vi "Felix Event FSM Producer-Consumer Template.vi"() -> ()   [LabVIEW 2017]
uses:
  FSM Queue Datatype.ctl
panel:
  out "starat seq 2 argument":dbl
  in  "Seq 2 argument":dbl format="%#_13g"
  in  "Loop Back":bool
  in  "Skip Step 2":bool
  out "FSM State":string
  out "LED 2.3":bool
  out "LED 2.2":bool
  out "LED 2.1":bool
  out "LED 1.3":bool
  out "LED 1.2":bool
  out "LED 1.1":bool
  in  "Start Sequence 2":bool
  in  "Start Sequence 1":bool
  in  "stop":bool
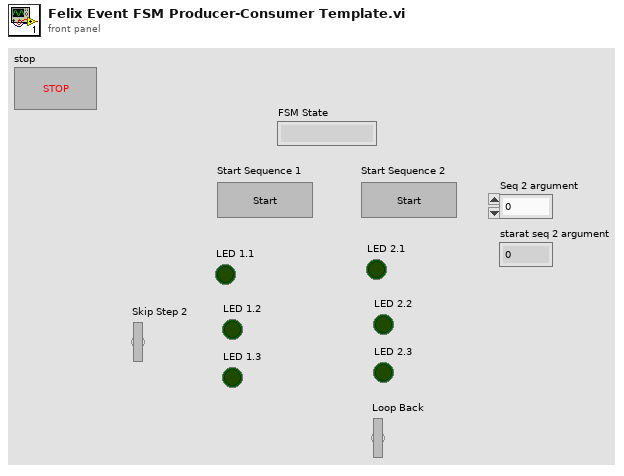
[diagram p1: front panel]
types:
  T1 = cluster{"Variable 1":i32, "FSM State":string, "Loop Seq 2":bool}
  T2 = typedef "FSM Queue Datatype.ctl" = enum16{"INIT", "Start Seq 1", "Start Seq 2", "Set Seq 2 loop", "Exit"}
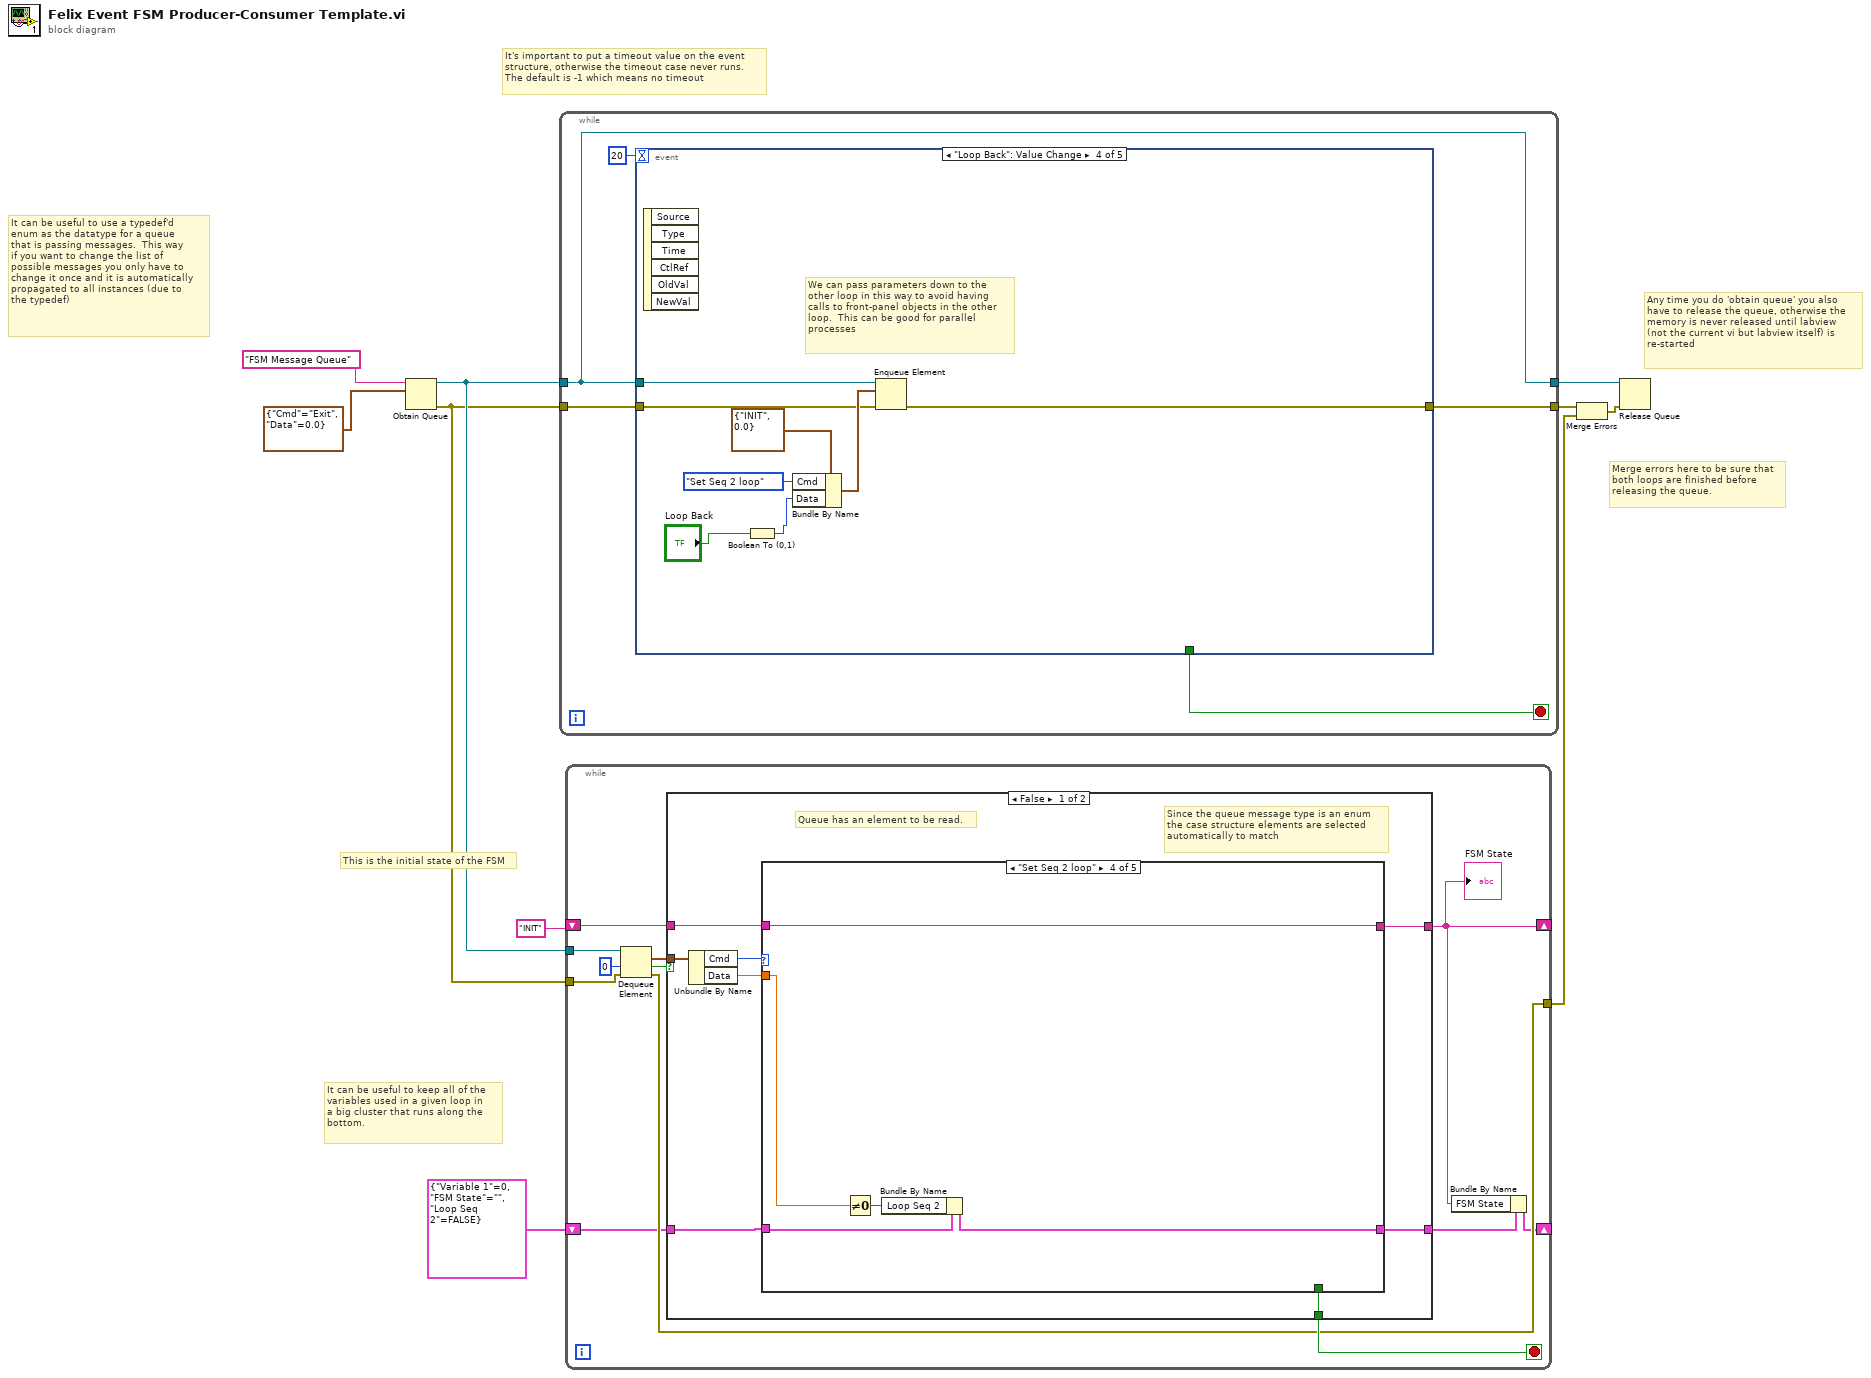
[diagram p0: block diagram]
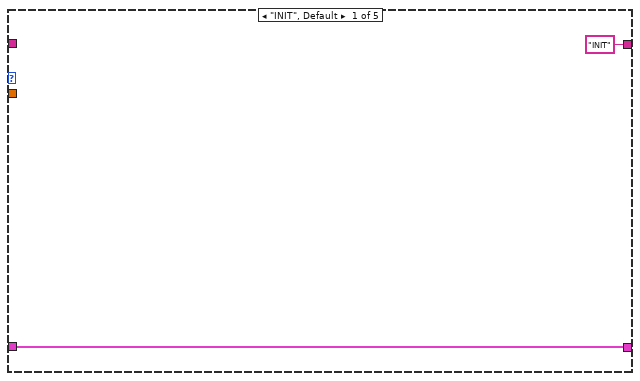
[diagram p2: hidden frame]
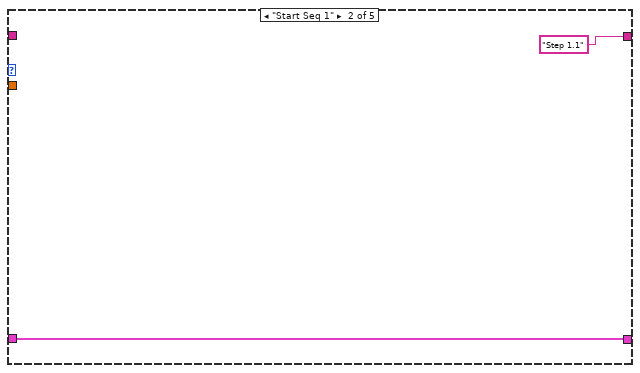
[diagram p3: hidden frame]
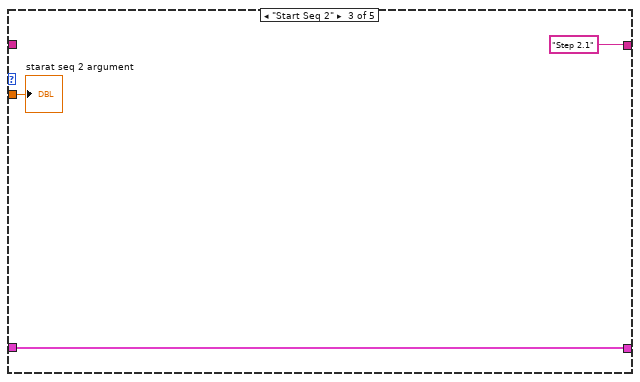
[diagram p4: hidden frame]
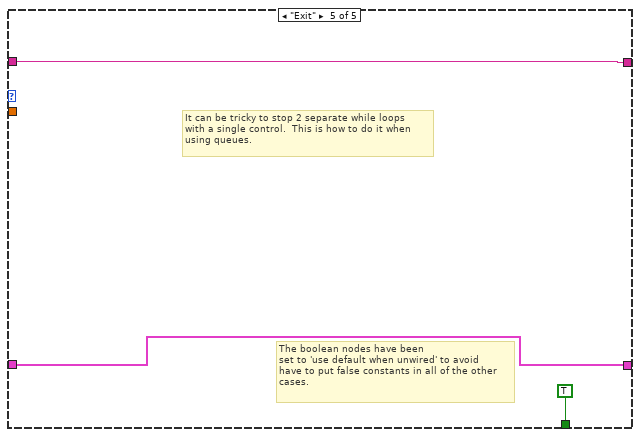
[diagram p5: hidden frame]
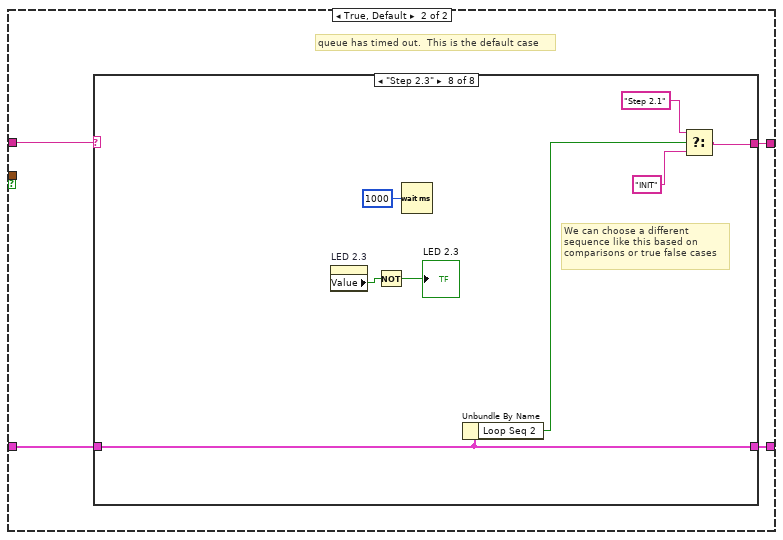
[diagram p6: hidden frame]
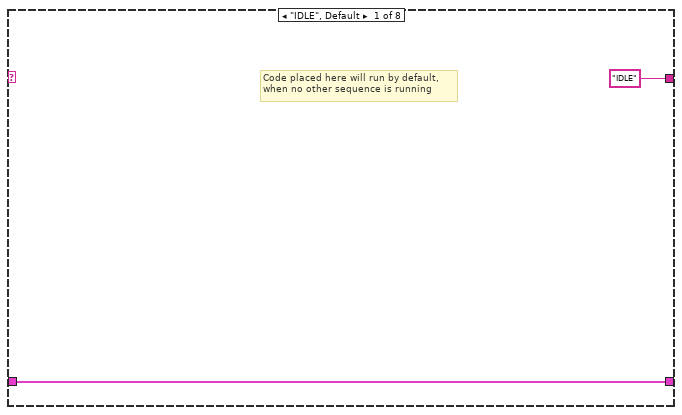
[diagram p7: hidden frame]
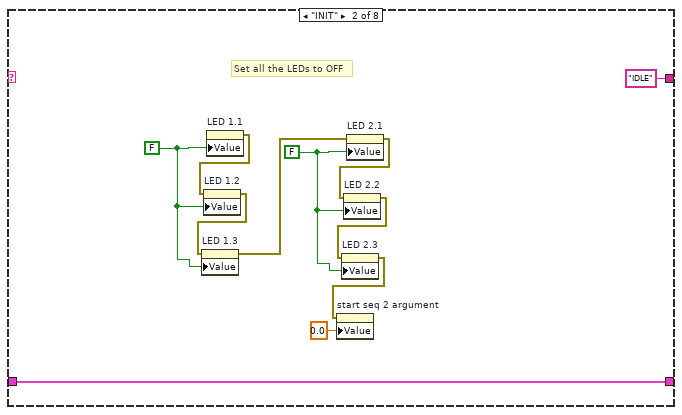
[diagram p8: hidden frame]
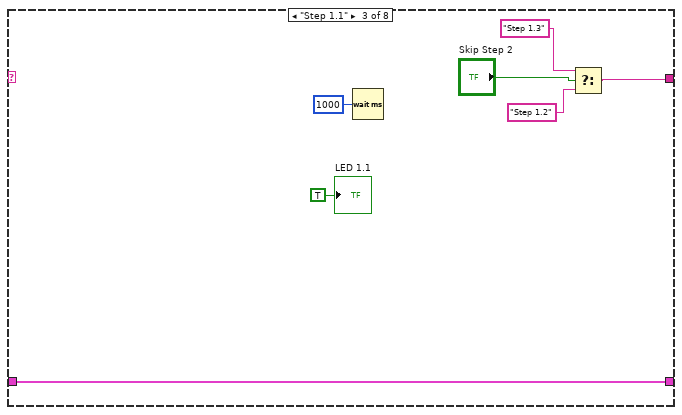
[diagram p9: hidden frame]
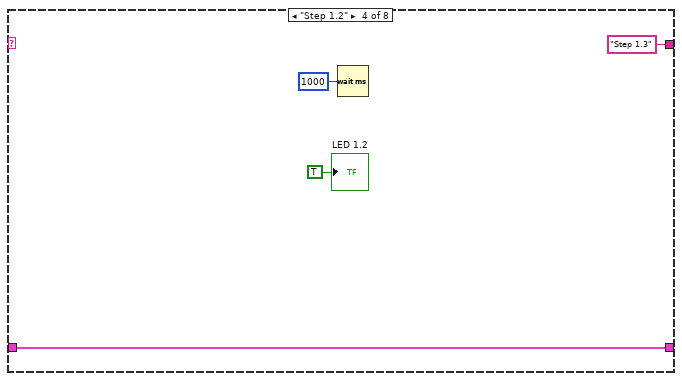
[diagram p10: hidden frame]
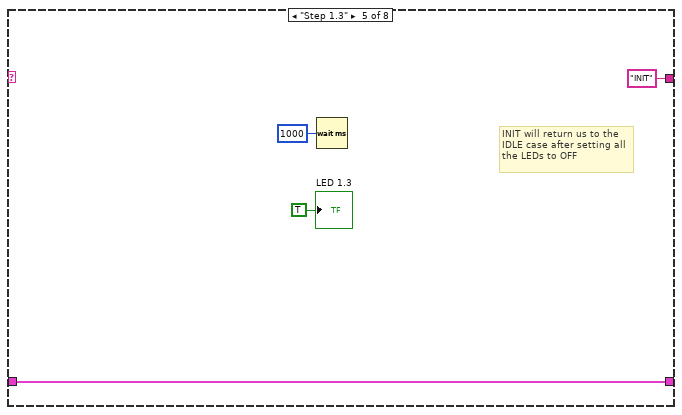
[diagram p11: hidden frame]
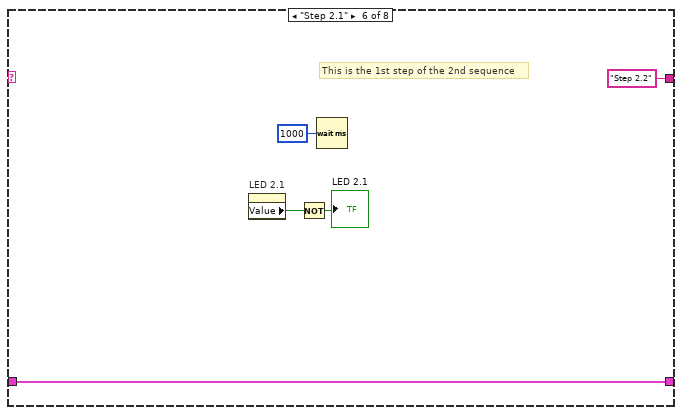
[diagram p12: hidden frame]
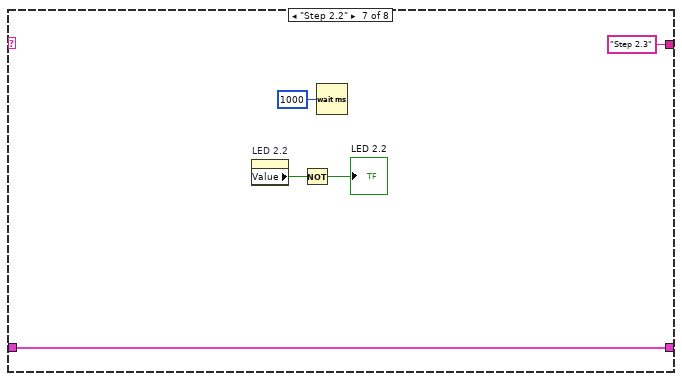
[diagram p13: hidden frame]
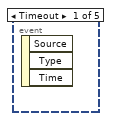
[diagram p14: hidden frame]
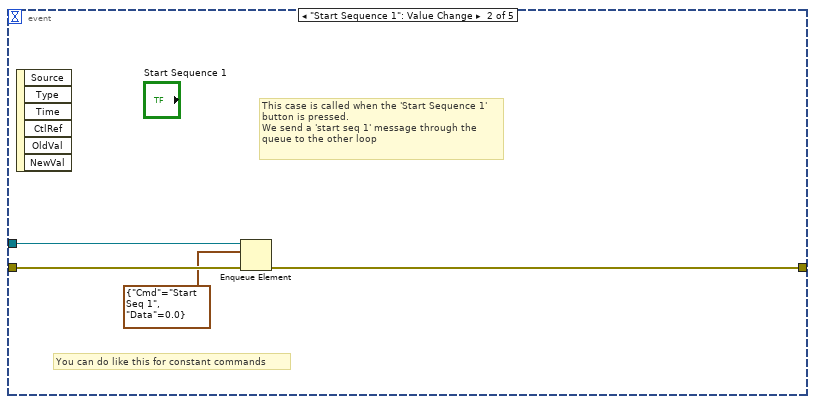
[diagram p15: hidden frame]
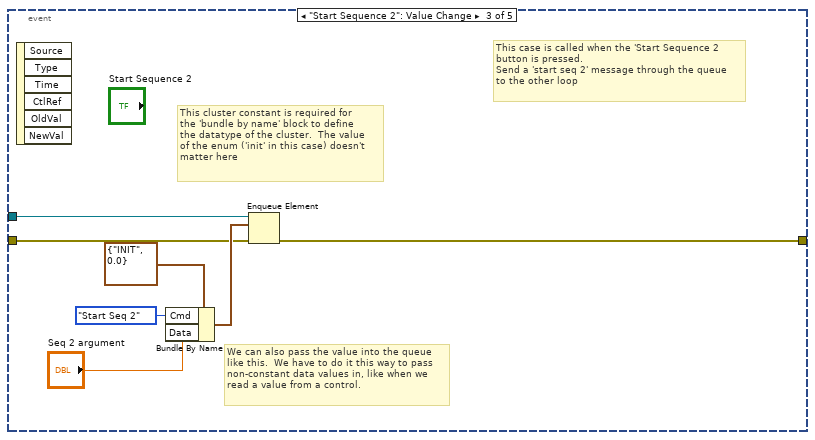
[diagram p16: hidden frame]
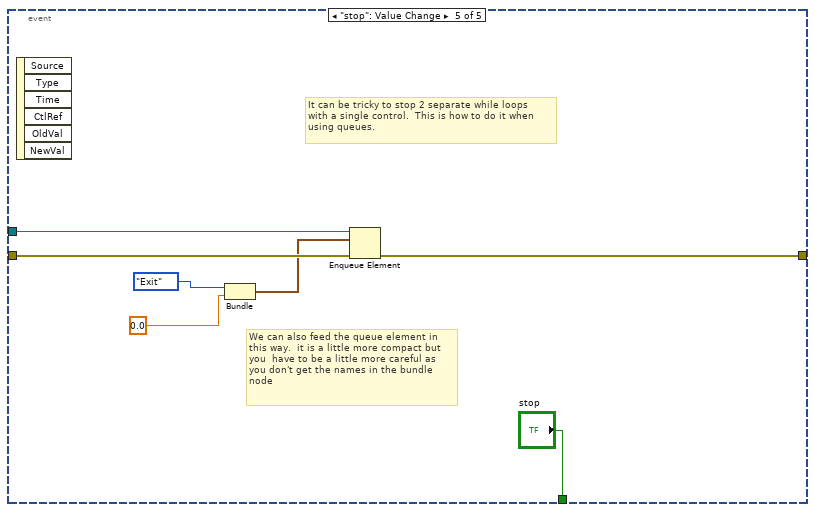
[diagram p17: hidden frame]
diagram:
  # "It can be useful to keep all of the \nvariables used in a given loop in\na big cluster that runs along the \nbottom."
  # "Merge errors here to be sure that\nboth loops are finished before\nreleasing the queue."
  # "Any time you do 'obtain queue' you also\nhave to release the queue, otherwise the\nmemory is never released until labview \n(not the current vi but labview itself) is\nre-started"
  # "It can be useful to use a typedef'd\nenum as the datatype for a queue\nthat is passing messages.  This way\nif you want to change the list of \npossible messages you only have to \nchange it once and it is automatically\npropagated to all instances (due to\nthe typedef)"
  # "This is the initial state of the FSM"
  # "It's important to put a timeout value on the event\nstructure, otherwise the timeout case never runs. \nThe default is -1 which means no timeout"
  n1 = Obtain Queue(name (unnamed)="FSM Message Queue", element data type=cluster{"Cmd":T2, "Data":dbl} {"Cmd"=enum."Exit", "Data"=0.0}) -> (queue out=w6:refnum<queue>, error out=w5:errorcluster)  [unwired: 3 in, 1 out]
  n2 = while {
    tunnel: w6 -> [w13]
    tunnel: w5 -> [w14]
    tunnel: [w13] -> w7
    tunnel: [w11] -> w4
    stop <- w12 stop-if-true
    n3 = event shown="[3] \"Loop Back\": Value Change" {
      selector: _ -> [_ _ _ _ _]
      dyn-events: _ -> [_ _ _ _ _]
      timeout: 20 -> [_ _ _ _ _]
      tunnel: w13 -> [_ w19 w23 w31 w40]
      tunnel: w14 -> [_ w18 w22 w30 w39]
      tunnel: [_ _ _ _ "stop"] -> w12
      tunnel: [_ w16 w20 w29 w38] -> w11
      event Timeout {
        n4 = event-data() -> ()  [unwired: 1 in, 3 out]
      }
      event "Start Sequence 1": Value Change {
        # "You can do like this for constant commands"
        # "This case is called when the 'Start Sequence 1'\nbutton is pressed.\nWe send a 'start seq 1' message through the\nqueue to the other loop"
        n5 = event-data() -> ()  [unwired: 1 in, 6 out]
        n6 = Enqueue Element(queue=w19, element=cluster{"Cmd":T2, "Data":dbl} {"Cmd"=enum."Start Seq 1", "Data"=0.0}, error in (no error)=w18) -> (error out=w16:errorcluster)  [unwired: 1 in, 2 out]
      }
      event "Start Sequence 2": Value Change {
        # "This cluster constant is required for\nthe 'bundle by name' block to define\nthe datatype of the cluster.  The value\nof the enum ('init' in this case) doesn't\nmatter here"
        # "We can also pass the value into the queue\nlike this.  We have to do it this way to pass\nnon-constant data values in, like when we\nread a value from a control."
        # "This case is called when the 'Start Sequence 2\nbutton is pressed.\nSend a 'start seq 2' message through the queue\nto the other loop"
        n7 = event-data() -> ()  [unwired: 1 in, 6 out]
        n8 = Bundle By Name(cluster=cluster{"Cmd":T2, "Data":dbl} {"Cmd"=enum."INIT", "Data"=0.0} ("element"), "Cmd"=FSM_Queue_Datatype."Start Seq 2", "Data"="Seq 2 argument") -> (w25:cluster{"Cmd":T2, "Data":dbl})
        n9 = Enqueue Element(queue=w23, element=w25, error in (no error)=w22) -> (error out=w20:errorcluster)  [unwired: 1 in, 2 out]
      }
      event "Loop Back": Value Change {
        # "We can pass parameters down to the \nother loop in this way to avoid having\ncalls to front-panel objects in the other\nloop.  This can be good for parallel \nprocesses"
        n10 = event-data() -> ()  [unwired: 1 in, 6 out]
        n11 = Boolean To (0,1)(Boolean="Loop Back") -> (0, 1=w27:i16)
        n12 = Bundle By Name(cluster=cluster{"Cmd":T2, "Data":dbl} {"Cmd"=enum."INIT", "Data"=0.0} ("element"), "Cmd"=FSM_Queue_Datatype."Set Seq 2 loop", "Data"=w27) -> (w33:cluster{"Cmd":T2, "Data":dbl})
        n13 = Enqueue Element(queue=w31, element=w33, error in (no error)=w30) -> (error out=w29:errorcluster)  [unwired: 1 in, 2 out]
      }
      event "stop": Value Change {
        # "It can be tricky to stop 2 separate while loops\nwith a single control.  This is how to do it when\nusing queues."
        # "We can also feed the queue element in\nthis way.  it is a little more compact but\nyou  have to be a little more careful as\nyou don't get the names in the bundle\nnode"
        n14 = event-data() -> ()  [unwired: 1 in, 6 out]
        n15 = Bundle("Cmd"=FSM_Queue_Datatype."Exit", "Data"=0.0) -> (w35:cluster{"Cmd":T2, "Data":dbl})  [unwired: 1 in]
        n16 = Enqueue Element(queue=w40, element=w35, error in (no error)=w39) -> (error out=w38:errorcluster)  [unwired: 1 in, 2 out]
      }
    }
  }
  n17 = while {
    shift-right: [w42] -> _
    shift-left: "INIT" -> [w53]
    tunnel: w6 -> [w50]
    tunnel: w5 -> [w49]
    tunnel: [w46] -> w3
    shift-right: [w43] -> _
    shift-left: T1 {"Variable 1"=0, "FSM State"="", "Loop Seq 2"=FALSE} -> [w45]
    stop <- w47 stop-if-true
    n18 = Dequeue Element(queue=w50, timeout in ms (-1)=0, error in (no error)=w49) -> (element=w48:cluster{"Cmd":T2, "Data":dbl}, timed out?=w52:bool, error out=w46:errorcluster)  [unwired: 1 out]
    n19 = case shown="False" w52 {
      tunnel: [w59 w80] -> w42
      tunnel: w53 -> [w56 w79]
      tunnel: w48 -> [w61 _]
      tunnel: [w58 _] -> w47
      tunnel: w45 -> [w55 w78]
      tunnel: [w54 w77] -> w44
      frame False {
        # "Since the queue message type is an enum\nthe case structure elements are selected\nautomatically to match"
        # "Queue has an element to be read."
        n20 = Unbundle By Name(w61) -> ("Cmd"=w60:T2, "Data"=w57:dbl)
        n21 = case shown="\"Set Seq 2 loop\"" w60 {
          tunnel: ["INIT" ("f") "Step 1.1" ("f") "Step 2.1" ("f") w69 w75] -> w59
          tunnel: [_ _ _ _ TRUE] -> w58
          tunnel: w57 -> [_ _ w67 w70 _]
          tunnel: w56 -> [_ _ _ w69 w75]
          tunnel: w55 -> [w62 w64 w66 w73 w74]
          tunnel: [w62 w64 w66 w72 w74] -> w54
          frame "INIT", Default {
          }
          frame "Start Seq 1" {
          }
          frame "Start Seq 2" {
            "starat seq 2 argument" <- w67
          }
          frame "Set Seq 2 loop" {
            n22 = Not Equal To 0?(x=w70) -> (x != 0?=w71:bool)
            n23 = Bundle By Name(cluster=w73, "Loop Seq 2"=w71) -> (w72:T1)
          }
          frame "Exit" {
            # "It can be tricky to stop 2 separate while loops\nwith a single control.  This is how to do it when\nusing queues."
            # "The boolean nodes have been\nset to 'use default when unwired' to avoid \nhave to put false constants in all of the other\ncases."
          }
        }
      }
      frame True, Default {
        # "queue has timed out.  This is the default case"
        n24 = case shown="\"Step 2.3\"" w79 {
          tunnel: ["IDLE" "IDLE" w97 "Step 1.3" "INIT" "Step 2.2" "Step 2.3" w124] -> w80
          tunnel: w78 -> [w81 w83 w94 w101 w105 w109 w114 w120]
          tunnel: [w81 w83 w94 w101 w105 w109 w114 w120] -> w77
          frame "IDLE", Default {
            # "Code placed here will run by default,\nwhen no other sequence is running"
          }
          frame "INIT" {
            w87 = FALSE ("LED 2.1")
            w92 = FALSE ("LED 2.1")
            # "Set all the LEDs to OFF"
            n25 = property on="LED 1.1" class="Bool (strict)"("Value"=w92) -> (error out=w91:errorcluster)  [unwired: 2 in, 1 out]
            n26 = property on="LED 1.2" class="Bool (strict)"(error in=w91, "Value"=w92) -> (error out=w90:errorcluster)  [unwired: 1 in, 1 out]
            n27 = property on="LED 1.3" class="Bool (strict)"(error in=w90, "Value"=w92) -> (error out=w86:errorcluster)  [unwired: 1 in, 1 out]
            n28 = property on="LED 2.1" class="Bool (strict)"(error in=w86, "Value"=w87) -> (error out=w88:errorcluster)  [unwired: 1 in, 1 out]
            n29 = property on="LED 2.2" class="Bool (strict)"(error in=w88, "Value"=w87) -> (error out=w89:errorcluster)  [unwired: 1 in, 1 out]
            n30 = property on="LED 2.3" class="Bool (strict)"(error in=w89, "Value"=w87) -> (error out=w85:errorcluster)  [unwired: 1 in, 1 out]
            n31 = property on="start seq 2 argument" class="DigNum (strict)"(error in=w85, "Value"=0.0 ("starat seq 2 argument")) -> ()  [unwired: 1 in, 2 out]
          }
          frame "Step 1.1" {
            n32 = Wait (ms)(milliseconds to wait=u32 1000) -> ()  [unwired: 1 out]
            n33 = Select(t="Step 1.3", s="Skip Step 2", f="Step 1.2") -> (s? t:f=w97:string)
            "LED 1.1" <- TRUE ("LED 1.1")
          }
          frame "Step 1.2" {
            n34 = Wait (ms)(milliseconds to wait=u32 1000) -> ()  [unwired: 1 out]
            "LED 1.2" <- TRUE ("LED 1.2")
          }
          frame "Step 1.3" {
            # "INIT will return us to the\nIDLE case after setting all\nthe LEDs to OFF"
            n35 = Wait (ms)(milliseconds to wait=u32 1000) -> ()  [unwired: 1 out]
            "LED 1.3" <- TRUE ("LED 1.3")
          }
          frame "Step 2.1" {
            # "This is the 1st step of the 2nd sequence"
            n36 = property on="LED 2.1" class="Bool (strict)"() -> ("Value"=w111:bool)  [unwired: 2 in, 2 out]
            n37 = Not(x=w111) -> (.not. x?=→"LED 2.1":bool)
            n38 = Wait (ms)(milliseconds to wait=u32 1000) -> ()  [unwired: 1 out]
          }
          frame "Step 2.2" {
            n39 = property on="LED 2.2" class="Bool (strict)"() -> ("Value"=w116:bool)  [unwired: 2 in, 2 out]
            n40 = Not(x=w116) -> (.not. x?=→"LED 2.2":bool)
            n41 = Wait (ms)(milliseconds to wait=u32 1000) -> ()  [unwired: 1 out]
          }
          frame "Step 2.3" {
            # "We can choose a different\nsequence like this based on\ncomparisons or true false cases"
            n42 = property on="LED 2.3" class="Bool (strict)"() -> ("Value"=w122:bool)  [unwired: 2 in, 2 out]
            n43 = Not(x=w122) -> (.not. x?=→"LED 2.3":bool)
            n44 = Wait (ms)(milliseconds to wait=u32 1000) -> ()  [unwired: 1 out]
            n45 = Unbundle By Name(w120) -> ("Loop Seq 2"=w119:bool)
            n46 = Select(t="Step 2.1", s=w119, f="INIT") -> (s? t:f=w124:string)
          }
        }
      }
    }
    "FSM State" <- w42
    n47 = Bundle By Name(cluster=w44, "FSM State"=w42) -> (w43:T1)
  }
  n48 = Merge Errors(w4, w3) -> (w2:errorcluster)
  n49 = Release Queue(queue=w7, error in (no error)=w2) -> ()  [unwired: 1 in, 3 out]
